vi "MainQueue Ref.vi"(6 "Write:T/Read:(F)":bool, 8 "error in":errorcluster, 11 "queue in":refnum<queue>) -> (0 "error out":errorcluster, 3 "queue out":refnum<queue>)   [LabVIEW 2022 SP3]
uses:
  Type Def/MainStates Cluster.ctl
  Type Def/MainStates.ctl
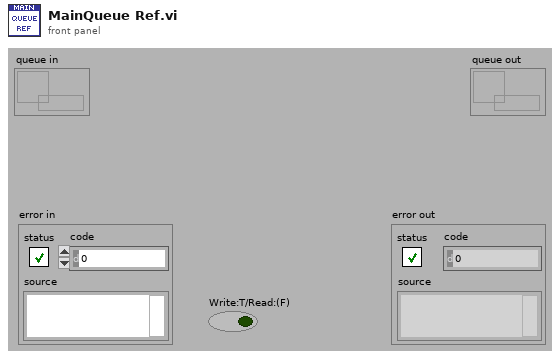
[diagram p1: front panel]
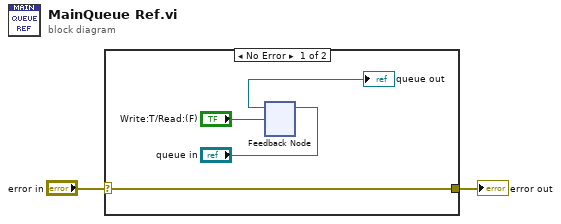
[diagram p0: block diagram]
diagram:
  n1 = case shown="No Error" "error in" {
    selector: "error in" -> [w6 w7]
    tunnel: [w6 w7] -> w1
    frame No Error {
      n2 = feedback-in #1("queue in", "Write:T/Read:(F)") -> ()
      n3 = feedback #1() -> (→"queue out":refnum<queue>)  [unwired: 1 in]
    }
    frame Error {
    }
  }
  "error out" <- w1
